vi "Write Has Value.vi"(8 "error in (no error)":errorcluster, 10 "Value Set":bool, 11 "Proto Type Common in":refnum<class "Proto Type Common.lvclass">) -> (0 "error out":errorcluster, 3 "Proto Type Common out":refnum<class "Proto Type Common.lvclass">)   [LabVIEW 2020]
uses:
  Proto Type Common.lvclass/Proto Type Common.ctl
  Proto Type Common.lvclass
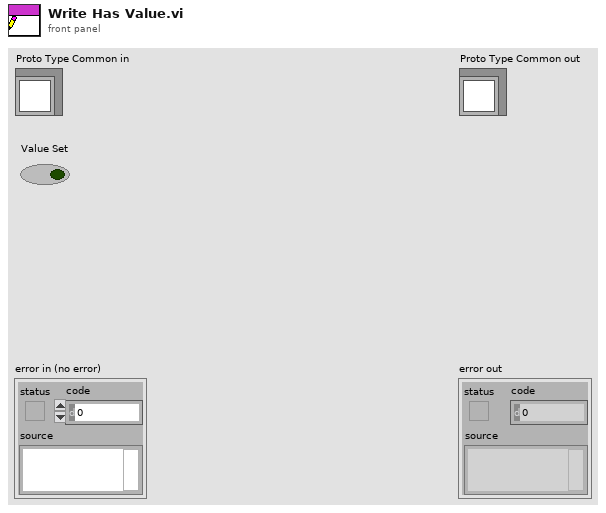
[diagram p1: front panel]
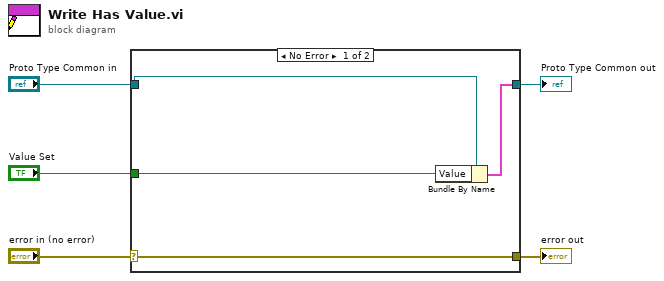
[diagram p0: block diagram]
diagram:
  n1 = case shown="No Error" "error in (no error)" {
    selector: "error in (no error)" -> [w9 w10]
    tunnel: [w9 w10] -> w4
    tunnel: [w7 w11] -> w2
    tunnel: "Proto Type Common in" -> [w8 w11]
    tunnel: "Value Set" -> [w6 _]
    frame No Error {
      n2 = Bundle By Name(cluster=w8, "Value"=w6) -> (w7:cluster{})
    }
    frame Error {
    }
  }
  "error out" <- w4
  "Proto Type Common out" <- w2
